vi "LabView laser project.vi"() -> ()   [LabVIEW 2020]
uses:
  <vilib>/Utility/error.llb/DialogType.ctl
  <vilib>/regexp/Match Regular Expression.xnode
panel:
  in  "laser voltage\nthreashold":dbl=2.5
  out "Numb of Samples":i32
  out "recieving\nprogress":dbl(slide) scale=0.0..1.0
  in  "aiming mode":bool
  out "sending progress":dbl(slide) scale=0.0..1.0
  out "end const. string":string
  in  "DAQ name":tag="Dev2"
  in  "Send":bool
  out "Max String length":i32
  out "sending":bool
  out "Data Rate":i32
  in  "Clear":bool
  out "end const. regex":string
  out "Resistor input":bool[](array[boolean])
  out "bits sent \nlast packet":dbl
  out "recieving":bool
  out "end constant":bool[](array[boolean])
  out "start constant":bool[](array[boolean])
  out "Laser output":bool[](array[boolean])
  in  "String Input":string
  out "String Output":string
  # "Local Variables"
  # "Debug output"
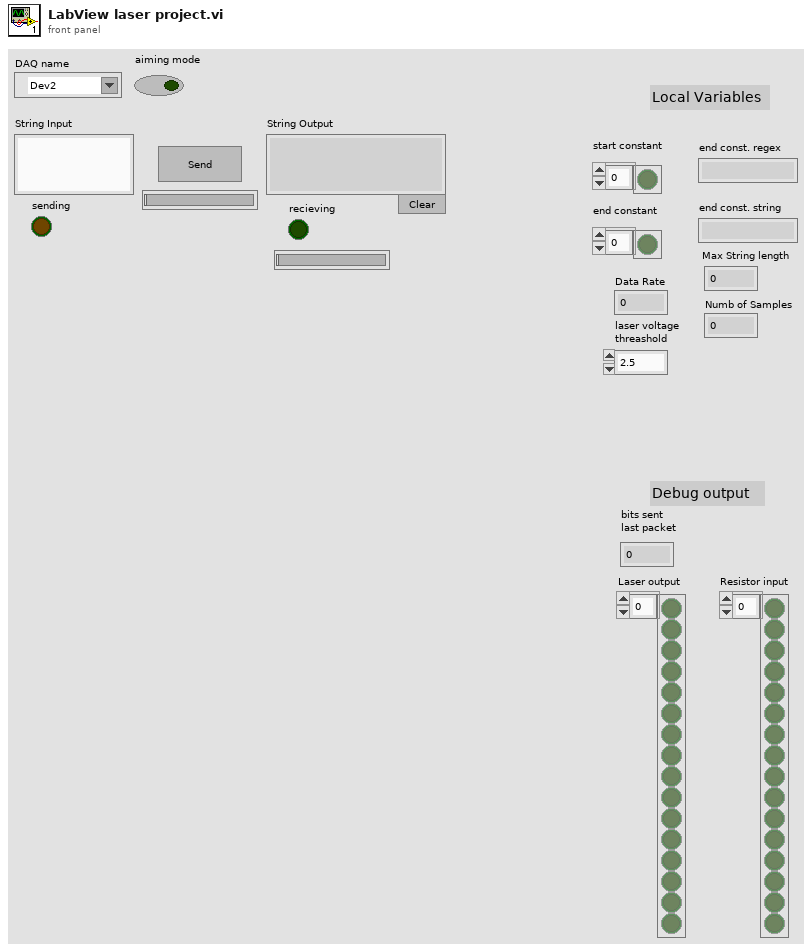
[diagram p1: front panel]
types:
  T1 = typedef "DialogType.ctl" = u16
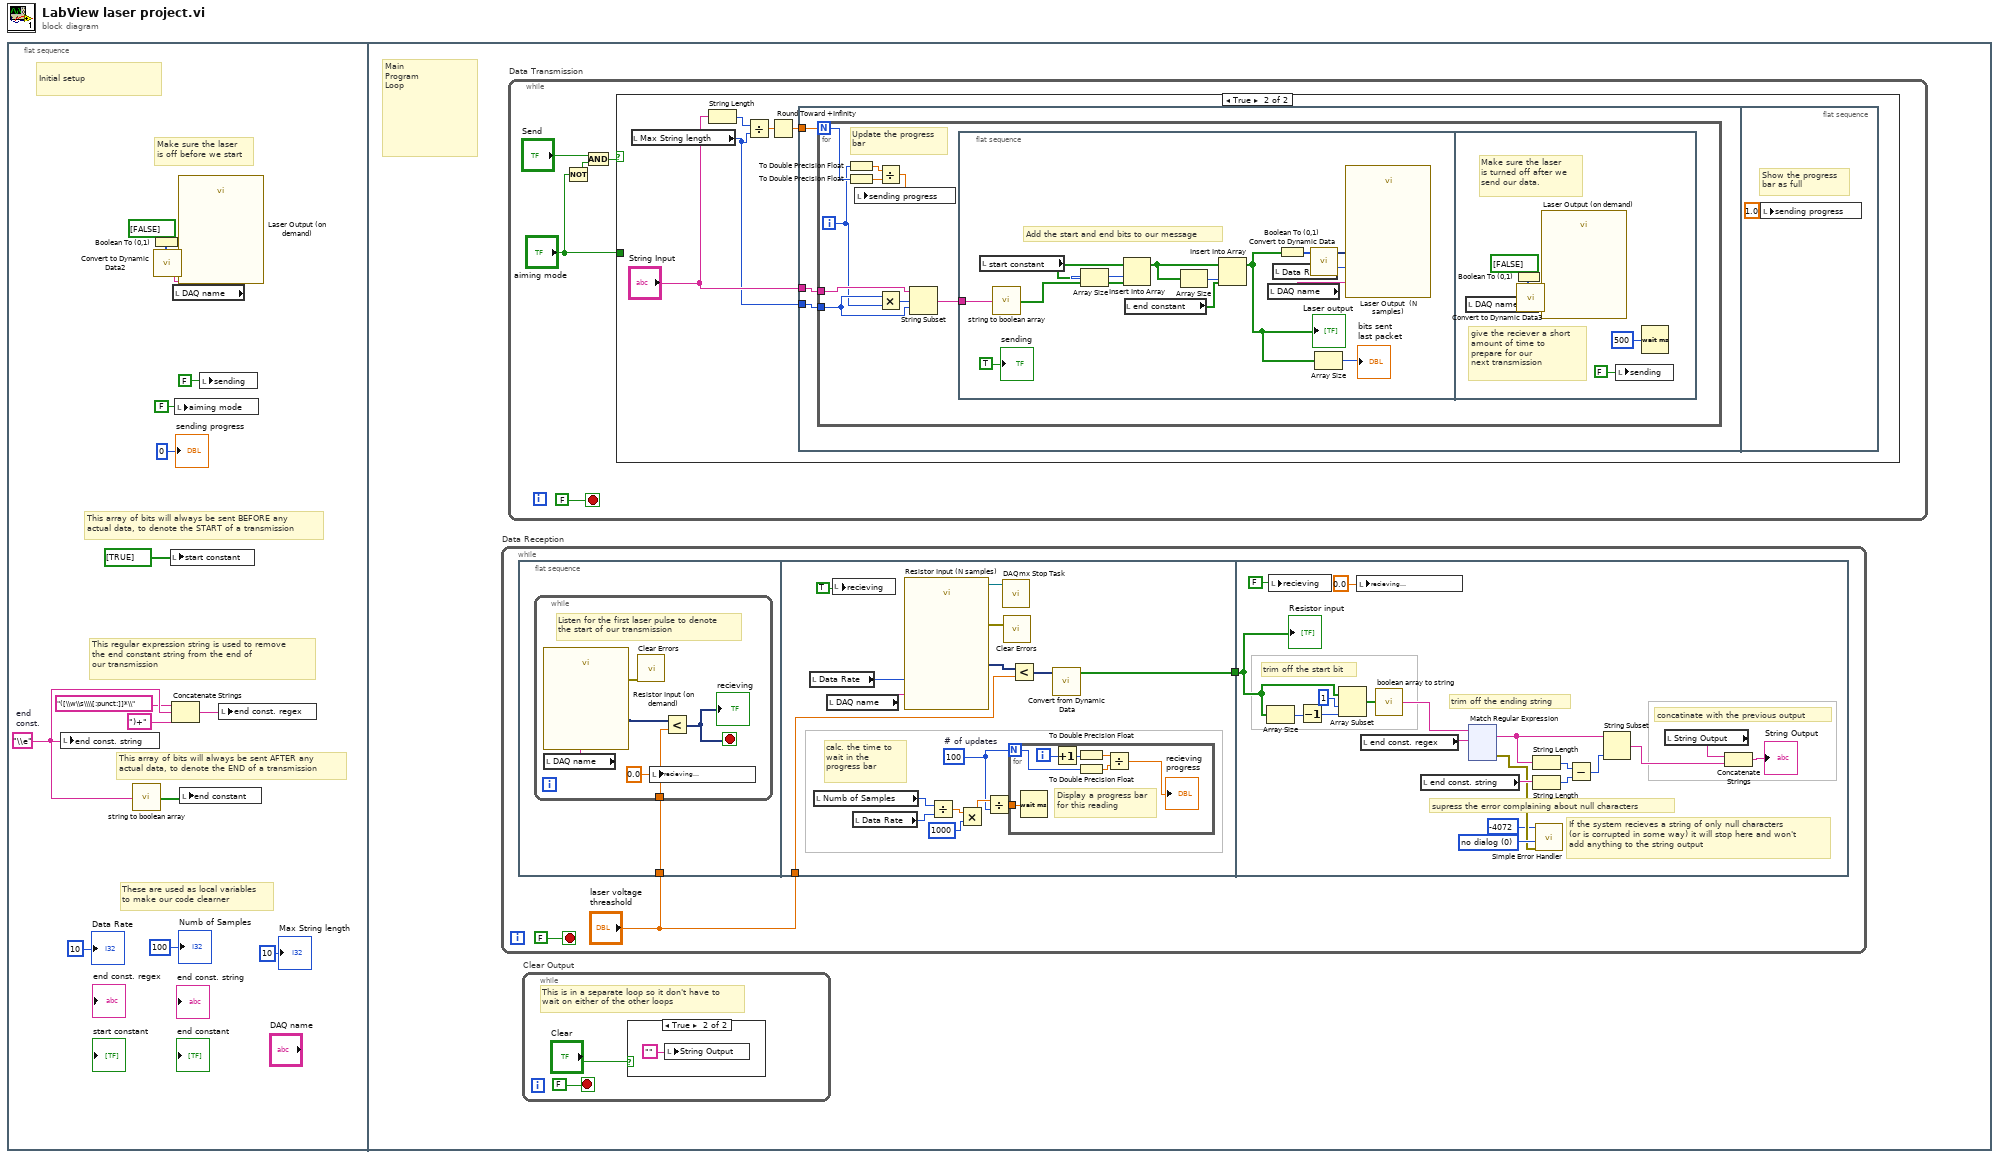
[diagram p0: block diagram]
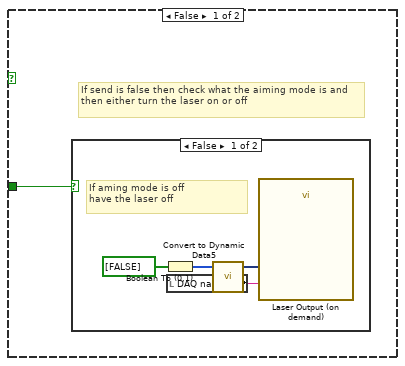
[diagram p3: hidden frame]
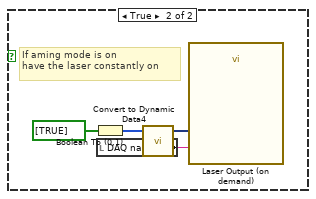
[diagram p4: hidden frame]
diagram:
  n1 = flat-sequence {
    frame #0 {
      w6 = "\\e"  # end  const.
      # "These are used as local variables\nto make our code clearner"
      # "Initial setup"
      # "This regular expression string is used to remove\nthe end constant string from the end of \nour transmission"
      # "This array of bits will always be sent AFTER any\nactual data, to denote the END of a transmission"
      # "This array of bits will always be sent BEFORE any\nactual data, to denote the START of a transmission"
      # "Make sure the laser\nis off before we start"
      n2 = local write "end const. string"(w6) -> ()
      n3 = call "string to boolean array.vi"("String Input"=w6) -> ("Boolean array"=w7:bool[])  [unwired: 4 in]
      n4 = Boolean To (0,1)(Boolean=bool[] [FALSE] ("array")) -> (0, 1=w16:i16[])
      n5 = call "Convert to Dynamic Data2"("Array"=w16) -> ("Dynamic Data Type"=w15:dynamicdata)  [unwired: 3 in]
      n6 = local write "start constant"(bool[] [TRUE] ("array")) -> ()
      n7 = Concatenate Strings("([\\w\\s\\\\[:punct:]]*\\", w6, ")+") -> (w8:string)
      n8 = local read "DAQ name"() -> (w12:tag)
      n9 = local write "aiming mode"(FALSE ("sending")) -> ()
      n10 = call "Laser Output (on demand)"("data"=w15, "device name"=w12) -> ()  [unwired: 16 in, 2 out]
      n11 = local write "end constant"(w7) -> ()
      n12 = local write "sending"(FALSE ("sending")) -> ()
      n13 = local write "end const. regex"(w8) -> ()
      "sending progress" <- u8 0 ("sending progress")
      "Data Rate" <- 10 ("Data Rate")
      "Max String length" <- 10 ("Max String length")
      "Numb of Samples" <- 100 ("Numb of Samples")
    }
    frame #1 {
      # "Main \nProgram\nLoop"
      n14 = while "Data Reception" {
        stop <- FALSE stop-if-true
        n15 = flat-sequence {
          tunnel: "laser voltage\nthreashold" -> [w23]
          tunnel: [w42] -> w21
          tunnel: "laser voltage\nthreashold" -> [w30]
          tunnel: w21 -> [w67]
          frame #0 {
            n16 = while {
              tunnel: w23 -> [w28]
              stop <- w25 stop-if-true
              # "Listen for the first laser pulse to denote\nthe start of our transmission"
              n17 = local read "DAQ name"() -> (w26:tag)
              n18 = call "Resistor Input (on demand)"("device name"=w26) -> ("data"=w27:dynamicdata, "error out"=w29:errorcluster)  [unwired: 16 in, 1 out]
              n19 = call <vilib>:"Clear Errors.vi"("error in (no error)"=w29) -> ()  [unwired: 5 in, 2 out]
              n20 = local write "recieving\nprogress"(0.0 ("recieving\nprogress")) -> ()
              n21 = Less?(x=w27, y=w28) -> (x < y?=w25:dynamicdata)
              "recieving" <- w25
            }
          }
          frame #1 {
            w33 = 100  # # of updates
            # "calc. the time to wait in the\nprogress bar"
            n22 = local read "Data Rate"() -> (w39:i32)
            n23 = local read "Numb of Samples"() -> (w35:i32)
            n24 = local read "DAQ name"() -> (w40:tag)
            n25 = local write "recieving"(TRUE) -> ()
            n26 = local read "Data Rate"() -> (w36:i32)
            n27 = call "Resistor Input (N samples)"("rate"=w39, "device name"=w40) -> ("task out"=w41:refnum<k21>, "data"=w43:dynamicdata, "error out"=w44:errorcluster)  [unwired: 14 in, 1 out]
            n28 = Divide(x=w35, y=w36) -> (x/y=w37:dbl)
            n29 = Multiply(x=w37, y=i16 1000) -> (x*y=w34:dbl)
            n30 = Divide(x=w34, y=w33) -> (x/y=w38:dbl)
            n31 = call <vilib>:"DAQmx Stop Task.vi"("task/channels in"=w41) -> ()  [unwired: 13 in, 2 out]
            n32 = call <vilib>:"Clear Errors.vi"("error in (no error)"=w44) -> ()  [unwired: 5 in, 2 out]
            n33 = for {
              N: w33 -> [w49]
              tunnel: w38 -> [w46]
              i -> [w48]
              # "Display a progress bar for this reading"
              n34 = Wait (ms)(milliseconds to wait=w46) -> ()  [unwired: 1 out]
              n35 = Increment(x=w48) -> (x+1=w47:i32)
              n36 = To Double Precision Float(number=w47) -> (double precision float=w51:dbl)
              n37 = To Double Precision Float(number=w49) -> (double precision float=w50:dbl)
              n38 = Divide(x=w51, y=w50) -> (x/y=→"recieving\nprogress":dbl)
            }
            n39 = Less?(x=w43, y=w30) -> (x < y?=w31:dynamicdata)
            n40 = call "Convert from Dynamic Data"("Dynamic Data Type"=w31) -> ("Array"=w42:bool[])  [unwired: 3 in]
          }
          frame #2 {
            w55 = T1 0 items=["no dialog", "OK message", "continue or stop message", "OK message + warnings", "continue/stop + warnings"] ("type of dialog (OK msg:1)")
            # "If the system recieves a string of only null characters \n(or is corrupted in some way) it will stop here and won't\nadd anything to the string output"
            # "supress the error complaining about null characters"
            # "concatinate with the previous output"
            # "trim off the ending string"
            # "trim off the start bit"
            n41 = Array Size(array=w67) -> (size(s)=w69:i32)
            n42 = local write "recieving"(FALSE) -> ()
            n43 = Decrement(x=w69) -> (x-1=w68:i32)
            n44 = Array Subset(array=w67, index=1, length=w68) -> (w66:bool[])
            n45 = local write "recieving\nprogress"(0.0 ("recieving\nprogress")) -> ()
            n46 = local read "end const. regex"() -> (w71:string)
            n47 = call "boolean array to string.vi"("Boolean array Input"=w66) -> ("String Output"=w56:string)  [unwired: 4 in]
            n48 = local read "end const. string"() -> (w62:string)
            n49 = xnode "Match Regular Expression"("input string"=w56, "regular expression"=w71) -> ("whole match"=w63:string, "error out"=w54:errorcluster)  [unwired: 4 in, 3 out]
            n50 = String Length(string=w63) -> (length=w60:i32)
            n51 = String Length(string=w62) -> (length=w59:i32)
            n52 = call <vilib>:"Simple Error Handler.vi"("error code (no error:0)"=-4072, "type of dialog (OK msg:1)"=w55, "error in (no error)"=w54) -> ()  [unwired: 2 in, 5 out]
            n53 = Subtract(x=w60, y=w59) -> (x-y=w58:i32)
            n54 = String Subset(string=w63, length (rest)=w58) -> (substring=w61:string)  [unwired: 1 in]
            n55 = local read "String Output"() -> (w64:string)
            n56 = Concatenate Strings(w64, w61) -> (→"String Output":string)
            "Resistor input" <- w67
          }
        }
      }
      n57 = while "Data Transmission" {
        stop <- FALSE stop-if-true
        n58 = Not(x="aiming mode") -> (.not. x?=w188:bool)
        n59 = And(x="Send", y=w188) -> (x .and. y?=w189:bool)
        n60 = case shown="True" w189 {
          tunnel: "aiming mode" -> [w192 _]
          frame False {
            # "If send is false then check what the aiming mode is and then either turn the laser on or off"
            n61 = case shown="False" w192 {
              frame False {
                # "If aming mode is off\nhave the laser off"
                n62 = Boolean To (0,1)(Boolean=bool[] [FALSE] ("array")) -> (0, 1=w193:i16[])
                n63 = local read "DAQ name"() -> (w196:tag)
                n64 = call "Convert to Dynamic Data5"("Array"=w193) -> ("Dynamic Data Type"=w194:dynamicdata)  [unwired: 3 in]
                n65 = call "Laser Output (on demand)"("data"=w194, "device name"=w196) -> ()  [unwired: 16 in, 2 out]
              }
              frame True {
                # "If aming mode is on\nhave the laser constantly on"
                n66 = Boolean To (0,1)(Boolean=bool[] [TRUE] ("array")) -> (0, 1=w197:i16[])
                n67 = local read "DAQ name"() -> (w199:tag)
                n68 = call "Convert to Dynamic Data4"("Array"=w197) -> ("Dynamic Data Type"=w200:dynamicdata)  [unwired: 3 in]
                n69 = call "Laser Output (on demand)"("data"=w200, "device name"=w199) -> ()  [unwired: 16 in, 2 out]
              }
            }
          }
          frame True {
            n70 = local read "Max String length"() -> (w204:i32)
            n71 = String Length(string="String Input") -> (length=w203:i32)
            n72 = Divide(x=w203, y=w204) -> (x/y=w202:dbl)
            n73 = Round Toward +Infinity(x=w202) -> (ceil(x): smallest int >= x=w201:dbl)
            n74 = flat-sequence {
              tunnel: "String Input" -> [w208]
              tunnel: w204 -> [w207]
              tunnel: w201 -> [w206]
              frame #0 {
                n75 = for {
                  N: w206 -> [w211]
                  tunnel: w208 -> [w217]
                  tunnel: w207 -> [w214]
                  i -> [w209]
                  # "Update the progress\nbar"
                  n76 = To Double Precision Float(number=w209) -> (double precision float=w212:dbl)
                  n77 = To Double Precision Float(number=w211) -> (double precision float=w210:dbl)
                  n78 = Divide(x=w212, y=w210) -> (x/y=w213:dbl)
                  n79 = local write "sending progress"(w213) -> ()
                  n80 = Multiply(x=w214, y=w209) -> (x*y=w215:i32)
                  n81 = String Subset(string=w217, offset (0)=w215, length (rest)=w214) -> (substring=w216:string)
                  n82 = flat-sequence {
                    tunnel: w216 -> [w220]
                    frame #0 {
                      # "Add the start and end bits to our message"
                      n83 = local read "start constant"() -> (w226:bool[])
                      n84 = call "string to boolean array.vi"("String Input"=w220) -> ("Boolean array"=w225:bool[])  [unwired: 4 in]
                      n85 = Array Size(array=w226) -> (size(s)=w231:i32)
                      n86 = Insert Into Array(array=w226, index=w231, new element=w225) -> (w224:bool[])
                      n87 = local read "end constant"() -> (w218:bool[])
                      n88 = Array Size(array=w224) -> (size(s)=w230:i32)
                      n89 = Insert Into Array(array=w224, index=w230, new element=w218) -> (w227:bool[])
                      "Laser output" <- w227
                      n90 = local read "DAQ name"() -> (w219:tag)
                      n91 = local read "Data Rate"() -> (w222:i32)
                      n92 = Boolean To (0,1)(Boolean=w227) -> (0, 1=w223:i16[])
                      n93 = call "Convert to Dynamic Data"("Array"=w223) -> ("Dynamic Data Type"=w229:dynamicdata)  [unwired: 3 in]
                      n94 = Array Size(array=w227) -> (size(s)=→"bits sent \nlast packet":i32)
                      n95 = call "Laser Output  (N samples)"("data"=w229, "rate"=w222, "device name"=w219) -> ()  [unwired: 15 in, 2 out]
                      "sending" <- TRUE ("sending")
                    }
                    frame #1 {
                      # "give the reciever a short \namount of time to \nprepare for our \nnext transmission"
                      # "Make sure the laser\nis turned off after we \nsend our data."
                      n96 = local read "DAQ name"() -> (w232:tag)
                      n97 = Boolean To (0,1)(Boolean=bool[] [FALSE] ("array")) -> (0, 1=w237:i16[])
                      n98 = call "Convert to Dynamic Data3"("Array"=w237) -> ("Dynamic Data Type"=w236:dynamicdata)  [unwired: 3 in]
                      n99 = call "Laser Output (on demand)"("data"=w236, "device name"=w232) -> ()  [unwired: 16 in, 2 out]
                      n100 = local write "sending"(FALSE ("sending")) -> ()
                      n101 = Wait (ms)(milliseconds to wait=u32 500) -> ()  [unwired: 1 out]
                    }
                  }
                }
              }
              frame #1 {
                # "Show the progress\nbar as full"
                n102 = local write "sending progress"(1.0 ("sending progress")) -> ()
              }
            }
          }
        }
      }
      n103 = while "Clear Output" {
        stop <- FALSE stop-if-true
        # "This is in a separate loop so it don't have to\nwait on either of the other loops"
        n104 = case shown="True" "Clear" {
          frame False {
          }
          frame True {
            n105 = local write "String Output"("") -> ()
          }
        }
      }
    }
  }
